vi "testRegUserEvent.vi"(8 "error in (no error)":errorcluster) -> (0 "error out":errorcluster)   [LabVIEW 2018]
doc: "Test the regUserEvent.vi."
uses:
  src/TcpServer/TcpServer.lvclass
  src/TcpServerCmd/typedef/ackTypeDef.ctl
  src/TcpServer/TcpServer.lvclass/TcpServer.ctl
  src/TcpServerCmd/TcpServerCmd.lvclass/TcpServerCmd.ctl
  <vilib>/addons/_JKI Toolkits/Caraya/classes/Assert/Assert Equal Type_Variant.vi
  src/TcpServerCmd/TcpServerCmd.lvclass
  <vilib>/addons/_JKI Toolkits/Caraya/classes/Test/Test.lvclass
  <vilib>/addons/_JKI Toolkits/Caraya/classes/Assert/Assert.lvclass
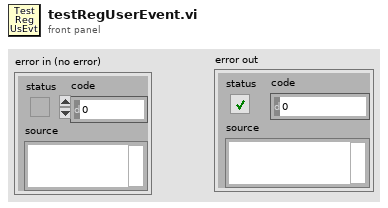
[diagram p1: front panel]
types:
  T1 = typedef "TcpServerCmd.lvclass/userEventTypeDef.ctl" = cluster{"CmdWrite":refnum<user-event>, "EvtWrite":refnum<user-event>, "CmdToServer":refnum<user-event>, "EvtToServer":refnum<user-event>}
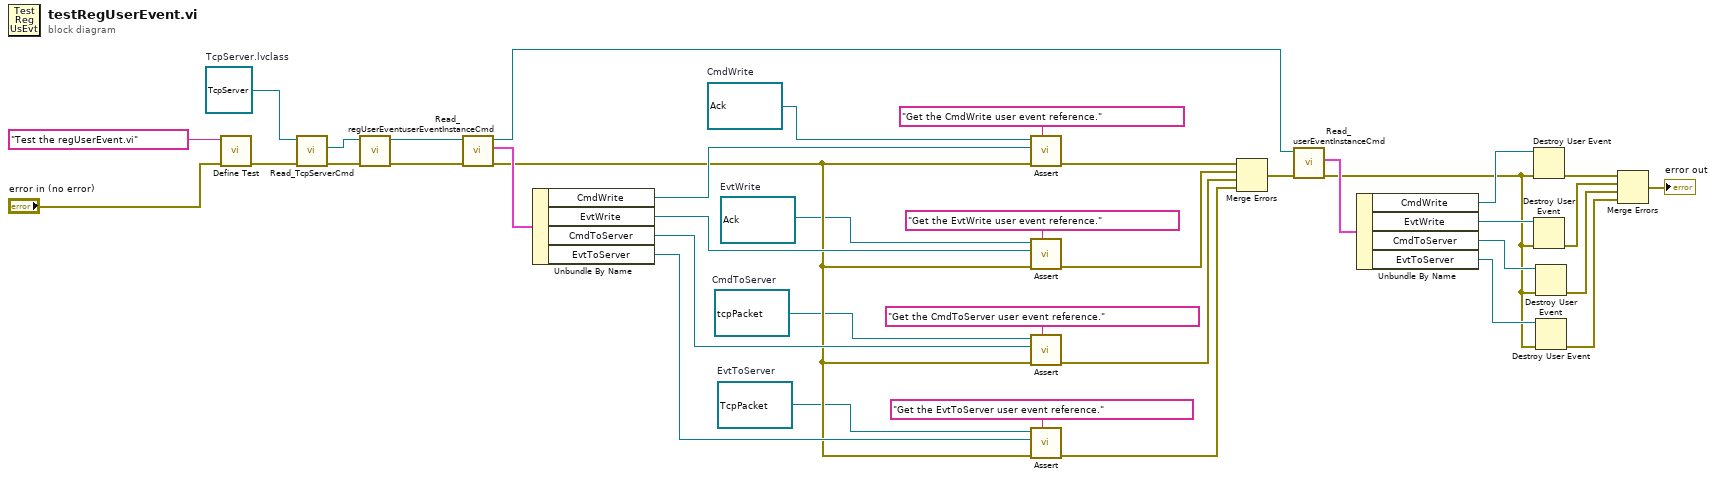
[diagram p0: block diagram]
diagram:
  w1 = refnum<user-event> refnum  # EvtToServer
  w2 = refnum<user-event> refnum  # CmdWrite
  w3 = refnum<user-event> refnum  # CmdToServer
  w4 = refnum<user-event> refnum  # EvtWrite
  w34 = refnum<class "TcpServer.lvclass"> refnum  # TcpServer.lvclass
  n1 = call <vilib>:"Define Test.vi"("error in (no error)"="error in (no error)", "Label (VI Title)"="Test the regUserEvent.vi") -> ("error out"=w38:errorcluster)  [unwired: 9 in]
  n2 = call "Read_TcpServerCmd.vi"("error in (no error)"=w38, "TcpServer in"=w34) -> ("error out"=w33:errorcluster, "TcpServerCmd.lvclass"=w32:refnum<class "TcpServerCmd.lvclass">)  [unwired: 7 in, 1 out]
  n3 = call "regUserEvent.vi"("error in (no error)"=w33, "tcpServerCmd in"=w32) -> ("error out"=w30:errorcluster, "tcpServerCmd out"=w31:refnum<class "TcpServerCmd.lvclass">)  [unwired: 8 in]
  n4 = call "Read_userEventInstanceCmd.vi"("error in (no error)"=w30, "TcpServerCmd in"=w31) -> ("error out"=w16:errorcluster, "userEventInstance"=w29:T1, "TcpServerCmd out"=w20:refnum<class "TcpServerCmd.lvclass">)  [unwired: 7 in]
  n5 = Unbundle By Name(w29) -> ("CmdWrite"=w28:refnum<user-event>, "EvtWrite"=w22:refnum<user-event>, "CmdToServer"=w24:refnum<user-event>, "EvtToServer"=w23:refnum<user-event>)
  n6 = call-poly <vilib>:"Assert.vi"("Label"="Get the CmdWrite user event reference.", "error in (no error)"=w16, "Y"=w28, "X"=w2) -> ("error out"=w35:errorcluster)  [unwired: 7 in]
  n7 = call-poly <vilib>:"Assert.vi"("Label"="Get the EvtWrite user event reference.", "error in (no error)"=w16, "Y"=w22, "X"=w4) -> ("error out"=w19:errorcluster)  [unwired: 7 in]
  n8 = call-poly <vilib>:"Assert.vi"("Label"="Get the CmdToServer user event reference.", "error in (no error)"=w16, "Y"=w24, "X"=w3) -> ("error out"=w18:errorcluster)  [unwired: 7 in]
  n9 = call-poly <vilib>:"Assert.vi"("Label"="Get the EvtToServer user event reference.", "error in (no error)"=w16, "Y"=w23, "X"=w1) -> ("error out"=w17:errorcluster)  [unwired: 7 in]
  n10 = Merge Errors(w35, w19, w18, w17) -> (w21:errorcluster)
  n11 = call "Read_userEventInstanceCmd.vi"("error in (no error)"=w21, "TcpServerCmd in"=w20) -> ("error out"=w10:errorcluster, "userEventInstance"=w15:T1)  [unwired: 7 in, 1 out]
  n12 = Unbundle By Name(w15) -> ("CmdWrite"=w14:refnum<user-event>, "EvtWrite"=w13:refnum<user-event>, "CmdToServer"=w12:refnum<user-event>, "EvtToServer"=w11:refnum<user-event>)
  n13 = Destroy User Event(user event=w14, error in=w10) -> (error out=w9:errorcluster)
  n14 = Destroy User Event(user event=w13, error in=w10) -> (error out=w8:errorcluster)
  n15 = Destroy User Event(user event=w12, error in=w10) -> (error out=w7:errorcluster)
  n16 = Destroy User Event(user event=w11, error in=w10) -> (error out=w6:errorcluster)
  n17 = Merge Errors(w9, w8, w7, w6) -> (→"error out":errorcluster)
